vi "Generation Stream Control Core.vi"(0 "SPC":u8=1, 1 "input valid":bool, 2 "request state":T1, 3 "num samples":u64, 4 "initial padding":u64, 5 "final padding":u64, 7 "ready for output (T)":bool=TRUE, 8 "reset":bool, 9 "start trigger":bool) -> (10 "cache write index":u8, 11 "ready for start":bool, 12 "cache read count":u8, 13 "ready for input":bool, 14 "cache discard read elements":bool, 15 "output valid":bool, 16 "actual state":T1, 17 "samples transferred":u64, 18 "output buffer write index":u8, 19 "output buffer latch enable":bool)   [LabVIEW 2018, in "Streaming FPGA.lvlib"]
doc: "<B>General</B>\n\nThis VI controls the signal generation data flow with a state machine controller. This enables the control and monitoring of finite and continuous streams of data between nodes using 4-wire handshaking. This VI provides control signals for the data transfer, but it does not handle the data transfer itself.\n\n<B>Signals</B>\n\nThe stream is controlled by the <B>request state</B>, <B>num samples</B>, <B>initial padding</B>, <B>final padding</B> and <B>start trigger</B> inputs. The stream is monitored by the <B>actual state</B>, <B>ready for start</B> and <B>samples transferred</B> outputs.\n\nThe upstream node can provide data by setting the <B>input valid</B> input to true. The data provided by the upstream node is accepted if the <B>input valid</B> input is true and the <B>ready for input</B> output was true in the previous cycle. If the <B>ready for input</B> output was false in the previous cycle, then the <B>input valid</B> input and the data provided by the upstream node are ignored in the current cycle.\n\nThe <B>output valid</B> output is set to true when data is available. The downstream node should set the <B>ready for output</B> input to true when it is ready for data. If the <B>ready for output</B> input is true and the <B>output valid</B> output is also true, then the downstream node should accept the data provided. If the <B>ready for output</B> input is false or if the <B>output valid</B> output is false, then the downstream should ignore the data provided.\n\n<B>Data movement control signals</B>\n\nThe <B>SPC</B> input should be set to the number of samples per clock cycle used by the upstream and downstream nodes. This VI assumes that the caller VI has a <B>data in</B> data input and a <B>data out</B> data output which are arrays of <B>SPC</B> number of samples. This VI also assumes that the caller implements a cache register which is an array of 2*<B>SPC</B>-1 number of samples and an output register which is an array of <B>SPC</B> number of samples. In each cycle the caller VI should update these registers and the <B>data out</B> data output in the following way:\n- Take the cache register output array and replace a subset of this array starting from the <B>cache write index</B> index using the <B>data in</B> data input as the new subarray if the <B>cache write index</B> output is between 0 and <B>SPC</B>-1. If the <B>cache write index</B> output is bigger than or equal to <B>SPC</B>, then do not replace elements. Denote the resulting array C1.\n- Create an array of 2*<B>SPC</B>-1 samples, denote this array C2. Copy the C1 array into C2 and rotate the C2 array by <B>cache read count</B> number of elements, so that the <B>cache read count</B>+n-th element in the C1 array becomes the n-th element in the C2 array.\n- Write the cache register by C2 if the <B>cache discard read elements</B> output is true, or by C1 if the <B>cache discard read elements</B> output is false.\n- Create an array of <B>SPC</B> padding samples, denote this array O1. Copy into O1 the first <B>cache read count</B> number of elements from the C1 array. Note that <B>cache read count</B> output can be between 0 and <B>SPC</B>.\n- Create an array of <B>SPC</B> padding samples, denote this array O2. Replace a subset of the O2 array starting from the <B>output buffer write index</B> index using O1 as the new subarray.\n- If the <B>output buffer latch enable</B> output is true, then write the output register by O2.\n- Write the <B>data out</B> data output by the output register output.\n\n<B>Detailed Operation</B>\n\nThere are two signal generation modes: finite or continuous mode. Each time a signal generation is started <B>initial padding</B> number of padding samples are provided to the downstream node first, followed by <B>num samples</B> samples (in case of finite mode) or an unspecified number of samples (in case of continuous mode) provided by the upstream node. At the end of the signal generation <B>final padding</B> number of padding samples are provided to the downstream node. A finite signal generation can be started by transitioning the state machine from the Idle state to the Finite Transfer state. A continuous signal generation can be started by transitioning the state machine from the Idle state to the Continuous state. Transitioning from the Idle state to the Finite Transfer or Continuous state does not start the signal generation immediately, when transitioning into these states the state machine always waits for a start trigger before starting the generation. The state machine sets the <B>ready for start</B> output to true when it is waiting for a start trigger in the next cycle (otherwise this output is false), the start trigger can be provided on the <B>start trigger</B> input by setting this input to true. The <B>start trigger</B> to <B>output valid</B> delay is 1 cycle. Note that this VI assumes that the signal generation should be continuous: during the signal generation if the <B>ready for output</B> input is true, but no data can be provided to the downstream node, the state machine aborts the signal generation and enters the Error state.\n\n<B>samples transferred</B> is updated with the number of upstream node provided samples accepted by the downstream node in the current cycle, that is, this counter does not include the number of initial/final padding samples provided to the downstream node.\n\nIn finite mode the state machine enters the Done state once the signal generation is finished. In the Done state the samples transferred continues to be reported until the user requests that the state machine return to Idle. A signal generation can be aborted by entering the Cancel state. When entering the Cancel state, the final padding samples are still provided to the downstream node (in case the generation was started), then the state machine transitions to the Not Ready state, then it can transition into the Idle state.\n\nThe data movement controls assume that an internal cache is used for storing samples provided by the upstream node. The upstream node is read in advance, samples stored in the internal cache are not flushed when a generation finishes, the samples remaining in the cache are returned during the next signal generation. The cache can be cleared by setting the <B>reset</B> input to true. This will also abort any ongoing signal generations but does not change the state of the internal state machine. In order to completely reset this VI set the <B>request state</B> input to Idle, set the <B>reset</B> input to true, wait until the <B>actual state</B> output indicates Idle, then set the <B>reset</B> input to false. Note that the upstream node is not read while this VI is in the Idle state.\n\n<b>States</b>\n\nThere are seven potential states for a stream defined by the Stream State.ctl typedef. All commanded states should be monitored from the controlling loop if it is important to ensure that the state is actually entered. The <B>request state</B> commands the stream into a state, and <B>actual state</B> reflects the current actual state.\n\nIdle - when the stream is ready to enter into an active state, it is in the Idle state. While it can be commanded directly to Idle from any state, it is advisable to do so with caution as samples abandoned in transfers may still need to be manually cleared out. It is generally safe to go directly from Done to Idle, and it is generally safe to request a transition from Not Ready to Idle. Other states may require further clean-up such as stopping/starting FIFOs or resetting other code under the command of the stream. Consider using Cancel instead (such as through the \"Stop Stream.vi\" in the host environment). While in Idle, <B>samples transferred</B> is reset to 0. \n\nFinite Transfer - Execute a transfer for the requested number of samples. Upon an orderly completion, this VI will automatically enter the Done state. If a stream underflows because the <B>ready for output</B> input is true, but no data can be provided to the downstream node, then the state machine enters the Error state.\n\nContinuous - Execute a transfer indefinitely. This state operates identically to the Finite Transfer state, but without regard to the <B>num samples</B> input.\n\nDone - In an orderly termination of a finite stream, the stream should end up here. At this point, <B>samples transferred</B> accurately reflects the terminal state of the transfer. The Done state should be exited by requesting Idle. Further active transfer modes (Finite or Continuous) will be ignored. This allows the host to distinguish between streams that are prematurely terminated (thus potentially requiring a flush of abandoned data) and ones that completed naturally.\n\nError - If the stream detects an unplanned interruption of the data, it enters the Error state. The only way to exit the Error state is to command the Generation Stream Control to Idle or Not Ready. When commanded to Idle or Not Ready, the Generation Stream Control advances first to Not Ready after the final padding samples are provided to the downstream node.\n\nNot Ready - In this state, the Generation Stream Control remains in the Not Ready state until the final padding samples are provided to the downstream node and the Generation Stream Control is commanded to Idle. This prevents starting a transfer in an obviously invalid state, and allows host control to wait until the not ready state is removed (such as by clearing out a FIFO under the streaming API's control).\n\nCancel - This state is indistinguishable from Error, but allows the controlling VI to know what condition caused the transfer to terminate."
uses:
  <instrlib>/_niInstr/Streaming/v1/Common/Stream State.ctl
  Streaming FPGA.lvlib
  <instrlib>/_niInstr/Streaming/v1/Common/niInstr Streaming v1 Common.lvlib
  <instrlib>/_niInstr/Basic Elements/v1/FPGA/niInstr Basic Elements v1 FPGA.lvlib
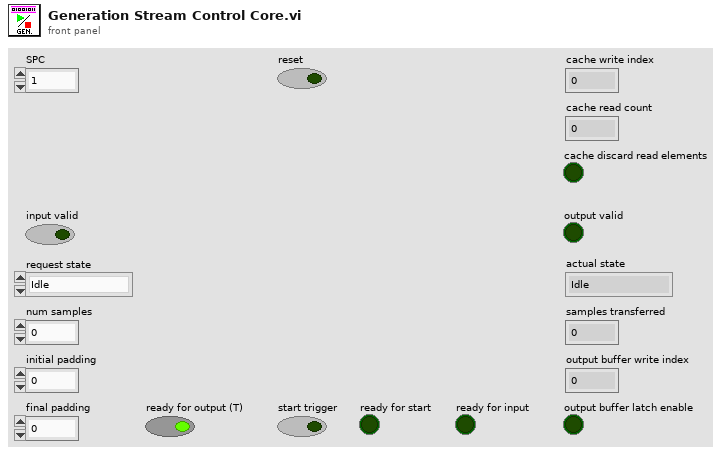
[diagram p1: front panel]
types:
  T1 = typedef "niInstr Streaming v1 Common.lvlib/Stream State.ctl" = enum8{"Idle", "Finite Transfer", "Continuous", "Done", "Error", "Not Ready", "Cancel"}
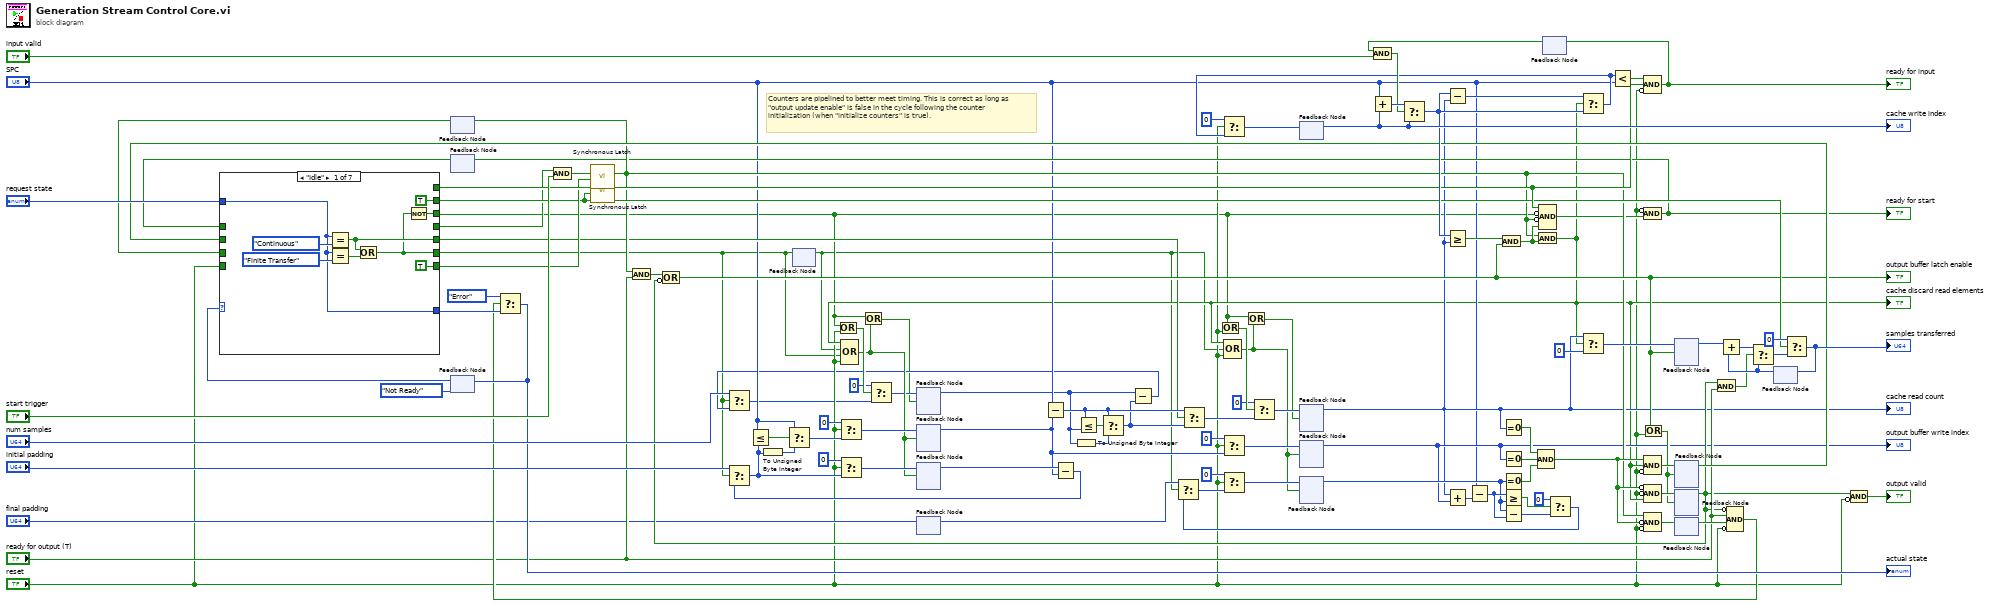
[diagram p0: block diagram]
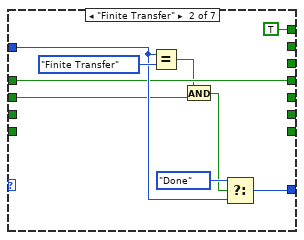
[diagram p2: hidden frame]
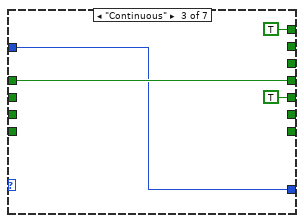
[diagram p3: hidden frame]
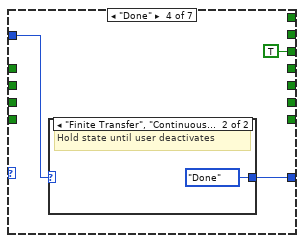
[diagram p4: hidden frame]
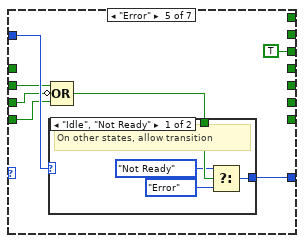
[diagram p6: hidden frame]
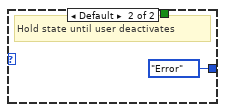
[diagram p7: hidden frame]
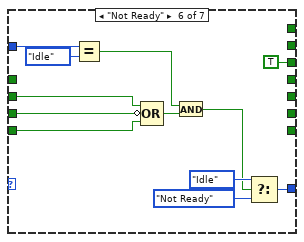
[diagram p8: hidden frame]
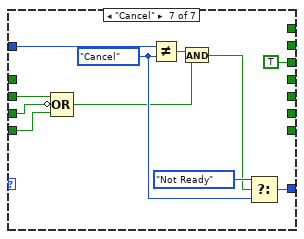
[diagram p9: hidden frame]
diagram:
  # "Counters are pipelined to better meet timing. This is correct as long as \"output update enable\" is false in the cycle following the counter initialization (when \"initialize counters\" is true)."
  n1 = feedback #1() -> (w85:bool)  [unwired: 1 in]
  n2 = feedback #2() -> (w84:bool)  [unwired: 1 in]
  n3 = feedback #3(Stream_State."Not Ready" ("request state")) -> (w56:T1)
  n4 = feedback #4() -> (w1:bool)  [unwired: 1 in]
  n5 = feedback #5() -> (w7:u64)  [unwired: 1 in]
  n6 = feedback #6() -> (w14:u8)  [unwired: 1 in]
  n7 = feedback #7() -> (w24:u64)  [unwired: 1 in]
  n8 = feedback #8() -> (w11:u64)  [unwired: 1 in]
  n9 = feedback-in #8("final padding") -> ()
  n10 = Subtract(x="SPC", y=w14) -> (x-y=w33:u8)
  n11 = Subtract(x=w24, y=w14) -> (x-y=w21:u64)
  n12 = To Unsigned Byte Integer(number=w7) -> (unsigned 8bit integer=w34:u8)
  n13 = Less Or Equal?(x=w33, y=w7) -> (x <= y?=w102:bool)
  n14 = Select(t=w33, s=w102, f=w34) -> (s? t:f=w26:u8)
  n15 = Subtract(x=w7, y=w26) -> (x-y=w6:u64)
  n16 = Select(t=u8 0, s="reset", f=w14) -> (s? t:f=w38:u8)
  n17 = feedback #9() -> (w104:u8)  [unwired: 1 in]
  "cache write index" <- w104
  n18 = feedback #10() -> (w25:u8)  [unwired: 1 in]
  "cache read count" <- w25
  n19 = feedback #11() -> (w27:u8)  [unwired: 1 in]
  "output buffer write index" <- w27
  n20 = feedback #12() -> (w95:u64)  [unwired: 1 in]
  n21 = Add(x="SPC", y=w104) -> (x+y=w105:u8)
  n22 = Add(x=w25, y=w27) -> (x+y=w100:u8)
  n23 = Subtract(x="SPC", y=w100) -> (x-y=w99:u8)
  n24 = Equal To 0?(x=w25) -> (x = 0?=w91:bool)
  n25 = Equal To 0?(x=w27) -> (x = 0?=w93:bool)
  n26 = Equal To 0?(x=w95) -> (x = 0?=w96:bool)
  n27 = Greater Or Equal?(x=w99, y=w95) -> (x >= y?=w97:bool)
  n28 = Subtract(x=w95, y=w99) -> (x-y=w98:u64)
  n29 = Compound Arithmetic op=AND(w91, w93, w96) -> (w54:bool)
  n30 = feedback #13() -> (w74:bool)  [unwired: 1 in]
  n31 = And(x=w74, y="input valid") -> (x .and. y?=w103:bool)
  n32 = Select(t=w105, s=w103, f=w104) -> (s? t:f=w83:u8)
  n33 = Subtract(x=w83, y=w25) -> (x-y=w101:u8)
  n34 = Greater Or Equal?(x=w83, y=w25) -> (x >= y?=w89:bool)
  n35 = Select(t=u64 0, s=w97, f=w98) -> (s? t:f=w30:u64)
  n36 = Select(t=w11, s=w1, f=w30) -> (s? t:f=w82:u64)
  n37 = Select(t=u64 0, s="reset", f=w82) -> (s? t:f=w81:u64)
  n38 = feedback #14() -> (w70:u8)  [unwired: 1 in]
  n39 = feedback #15() -> (w62:bool)  [unwired: 1 in]
  n40 = case shown="\"Idle\"" w56 {
    tunnel: "request state" -> [w116 w128 w130 w136 w145 w161 w173]
    tunnel: [w116 w126 w130 w135 w144 w159 w170] -> w52
    tunnel: [w113 _ _ _ _ _ _] -> w2
    tunnel: [w117 _ TRUE _ _ _ _] -> w31
    tunnel: [TRUE _ _ _ _ _ _] -> w57
    tunnel: w62 -> [_ w124 _ _ w142 w153 w167]
    tunnel: [_ TRUE TRUE _ _ _ _] -> w65
    tunnel: [TRUE _ _ _ _ _ _] -> w58
    tunnel: w85 -> [_ _ _ _ w141 w156 w166]
    tunnel: w84 -> [_ w123 w133 _ _ _ _]
    tunnel: [_ w123 w133 _ _ _ _] -> w46
    tunnel: [w112 _ _ TRUE TRUE TRUE TRUE] -> w8
    tunnel: "reset" -> [_ _ _ _ w140 w154 w165]
    frame "Idle" {
      n41 = Equal?(x=w116, y=Stream_State."Continuous") -> (x = y?=w117:bool)
      n42 = Equal?(x=w116, y=Stream_State."Finite Transfer") -> (x = y?=w118:bool)
      n43 = Or(x=w117, y=w118) -> (x .or. y?=w113:bool)
      n44 = Not(x=w113) -> (.not. x?=w112:bool)
    }
    frame "Finite Transfer" {
      n45 = Equal?(x=w128, y=Stream_State."Finite Transfer") -> (x = y?=w121:bool)
      n46 = And(x=w121, y=w124) -> (x .and. y?=w125:bool)
      n47 = Select(t=Stream_State."Done", s=w125, f=w128) -> (s? t:f=w126:T1)
    }
    frame "Continuous" {
    }
    frame "Done" {
      n48 = case shown="\"Finite Transfer\", \"Continuous\"" w136 {
        selector: w136 -> [w137 _]
        tunnel: [w137 Stream_State."Done" ("request state")] -> w135
        frame Default {
          # "On other states, allow transition"
        }
        frame "Finite Transfer", "Continuous" {
          # "Hold state until user deactivates"
        }
      }
    }
    frame "Error" {
      n49 = Compound Arithmetic op=OR(w142, invert w141, w140) -> (w139:bool)
      n50 = case shown="\"Idle\", \"Not Ready\"" w145 {
        tunnel: [w149 Stream_State."Error" ("request state")] -> w144
        tunnel: w139 -> [w147 _]
        frame "Idle", "Not Ready" {
          # "On other states, allow transition"
          n51 = Select(t=Stream_State."Not Ready", s=w147, f=Stream_State."Error" ("request state")) -> (s? t:f=w149:T1)
        }
        frame Default {
          # "Hold state until user deactivates"
        }
      }
    }
    frame "Not Ready" {
      n52 = Equal?(x=w161, y=Stream_State."Idle") -> (x = y?=w151:bool)
      n53 = Compound Arithmetic op=OR(w153, invert w156, w154) -> (w162:bool)
      n54 = And(x=w151, y=w162) -> (x .and. y?=w152:bool)
      n55 = Select(t=Stream_State."Idle" ("y"), s=w152, f=Stream_State."Not Ready") -> (s? t:f=w159:T1)
    }
    frame "Cancel" {
      w171 = Stream_State."Cancel" ("y")
      n56 = Compound Arithmetic op=OR(w167, invert w166, w165) -> (w163:bool)
      n57 = Not Equal?(x=w173, y=w171) -> (x != y?=w172:bool)
      n58 = And(x=w172, y=w163) -> (x .and. y?=w164:bool)
      n59 = Select(t=Stream_State."Not Ready", s=w164, f=w171) -> (s? t:f=w170:T1)
    }
  }
  n60 = And(x=w46, y="start trigger") -> (x .and. y?=w86:bool)
  n61 = call <instrlib>:"Synchronous Latch.vi"("clear"=w58, "set"=w86) -> ("out"=w44:bool)  [unwired: 9 in]
  n62 = feedback-in #1(w44) -> ()
  n63 = call <instrlib>:"Synchronous Latch.vi"("clear"=w57, "set"=w65) -> ("out"=w59:bool)  [unwired: 9 in]
  n64 = And(x=w44, y="ready for output (T)") -> (x .and. y?=w73:bool)
  n65 = Select(t="num samples", s=w2, f=w6) -> (s? t:f=w5:u64)
  n66 = Select(t="initial padding", s=w2, f=w21) -> (s? t:f=w16:u64)
  n67 = Less Or Equal?(x="SPC", y=w16) -> (x <= y?=w22:bool)
  n68 = To Unsigned Byte Integer(number=w16) -> (unsigned 8bit integer=w23:u8)
  n69 = Select(t="SPC", s=w22, f=w23) -> (s? t:f=w19:u8)
  n70 = feedback-in #4(w2) -> ()
  n71 = Or(x=w8, y="reset") -> (x .or. y?=w110:bool)
  n72 = Select(t=u64 0, s="reset", f=w16) -> (s? t:f=w36:u64)
  n73 = Select(t=u8 0, s="reset", f=w19) -> (s? t:f=w18:u8)
  n74 = Select(t=u64 0, s=w110, f=w5) -> (s? t:f=w4:u64)
  n75 = Select(t=w33, s=w31, f=w26) -> (s? t:f=w32:u8)
  n76 = Or(x=w8, y="reset") -> (x .or. y?=w111:bool)
  n77 = Select(t=u8 0, s=w111, f=w32) -> (s? t:f=w40:u8)
  n78 = Compound Arithmetic op=AND(w44, invert w54, invert "reset") -> (w53:bool)
  n79 = feedback #16() -> (w28:bool)  [unwired: 1 in]
  n80 = Compound Arithmetic op=OR(w73, invert w28) -> (w55:bool)
  "output buffer latch enable" <- w55
  n81 = And(x=w89, y=w55) -> (x .and. y?=w45:bool)
  n82 = And(x=w44, y=w45) -> (x .and. y?=w13:bool)
  "cache discard read elements" <- w13
  n83 = Compound Arithmetic op=OR(w13, w1, w2, "reset") -> (w9:bool)
  n84 = Or(x=w8, y=w9) -> (x .or. y?=w3:bool)
  n85 = feedback-in #5(w4, w3) -> ()
  n86 = feedback-in #6(w18, w9) -> ()
  n87 = feedback-in #7(w36, w9) -> ()
  n88 = Compound Arithmetic op=OR(w13, w1, "reset") -> (w20:bool)
  n89 = Or(x=w8, y=w20) -> (x .or. y?=w29:bool)
  n90 = feedback-in #10(w40, w29) -> ()
  n91 = feedback-in #11(w38, w20) -> ()
  n92 = feedback-in #12(w81, w20) -> ()
  n93 = Compound Arithmetic op=AND(w59, invert w8, invert w44, w45) -> (w43:bool)
  n94 = Select(t=w101, s=w13, f=w83) -> (s? t:f=w77:u8)
  n95 = Select(t=u8 0, s="reset", f=w77) -> (s? t:f=w107:u8)
  n96 = feedback-in #9(w107) -> ()
  n97 = Select(t=w25, s=w13, f=u8 0) -> (s? t:f=w72:u8)
  n98 = Less?(x=w77, y="SPC") -> (x < y?=w76:bool)
  n99 = Or(x=w55, y="reset") -> (x .or. y?=w60:bool)
  n100 = Compound Arithmetic op=AND(w76, w59, invert "reset") -> (w75:bool)
  "ready for input" <- w75
  n101 = feedback-in #13(w75) -> ()
  n102 = Compound Arithmetic op=AND(invert "reset", w43) -> (w42:bool)
  "ready for start" <- w42
  n103 = feedback-in #2(w42) -> ()
  n104 = Compound Arithmetic op=AND(w54, w13, invert "reset") -> (w61:bool)
  n105 = Compound Arithmetic op=AND(invert w54, invert "reset", w13) -> (w78:bool)
  n106 = feedback-in #14(w72, w55) -> ()
  n107 = feedback-in #15(w61, w60) -> ()
  n108 = feedback-in #16(w78, w60) -> ()
  n109 = feedback #17() -> (w48:bool)  [unwired: 1 in]
  n110 = feedback-in #17(w53) -> ()
  n111 = And(x=w28, y="ready for output (T)") -> (x .and. y?=w63:bool)
  n112 = Compound Arithmetic op=AND(invert w28, "ready for output (T)", w48, invert "reset") -> (w49:bool)
  n113 = Select(t=Stream_State."Error", s=w49, f=w52) -> (s? t:f=w50:T1)
  "actual state" <- w50
  n114 = feedback-in #3(w50) -> ()
  n115 = feedback #18() -> (w69:u64)  [unwired: 1 in]
  n116 = Add(x=w70, y=w69) -> (x+y=w71:u64)
  n117 = Select(t=w71, s=w63, f=w69) -> (s? t:f=w68:u64)
  n118 = Select(t=u64 0, s=w57, f=w68) -> (s? t:f=w67:u64)
  "samples transferred" <- w67
  n119 = feedback-in #18(w67) -> ()
  n120 = Compound Arithmetic op=AND(w28, invert "reset") -> (→"output valid":bool)
